vi "MWT_labview_final.vi"() -> ()   [LabVIEW 2019]
uses:
  <vilib>/BLE/type_def/connection_status_bundle.ctl
  <vilib>/BLE/type_def/address_type.ctl
  <vilib>/BLE/ble_functions/ble_write_by_service_characteristic_uint8array.vi
panel:
  out "characteristic value":u8[](array[numeric])
  in  "transmission inteveral (Seconds)":u8[](array[numeric]) format="%02x"
  out "Gradient graph":dbl(graph)
  out "Gradient":dbl
  out "VDD":dbl
  out "Temperature graph":dbl(graph)
  out "Temperature":dbl
  out "Rotation graph":dbl(graph)
  out "Rotation Speed":dbl
  in  "stop":bool
  out "Reading data":bool
  out "Connected":bool
  out "Device Name":string
  out "Handle table":string[][](array[string])
  out "Connection Status":T1={"MAC Address"="", "cnx handle"=0, "cnx flags"=0, "Address Type"=125, "Connection Interval (ms)"=125, "Timeout(ms)"=125, "Latency"=0, "bonding handle"=0} {"Address Type" items=["Public", "Random"]}
  out "Scanning":bool
  in  "COM Bluegiga in":refnum<visa-resource-name>="COM13"
  out "Devices":string[][](array[string])
  out "BLED112 Dongle Info":string
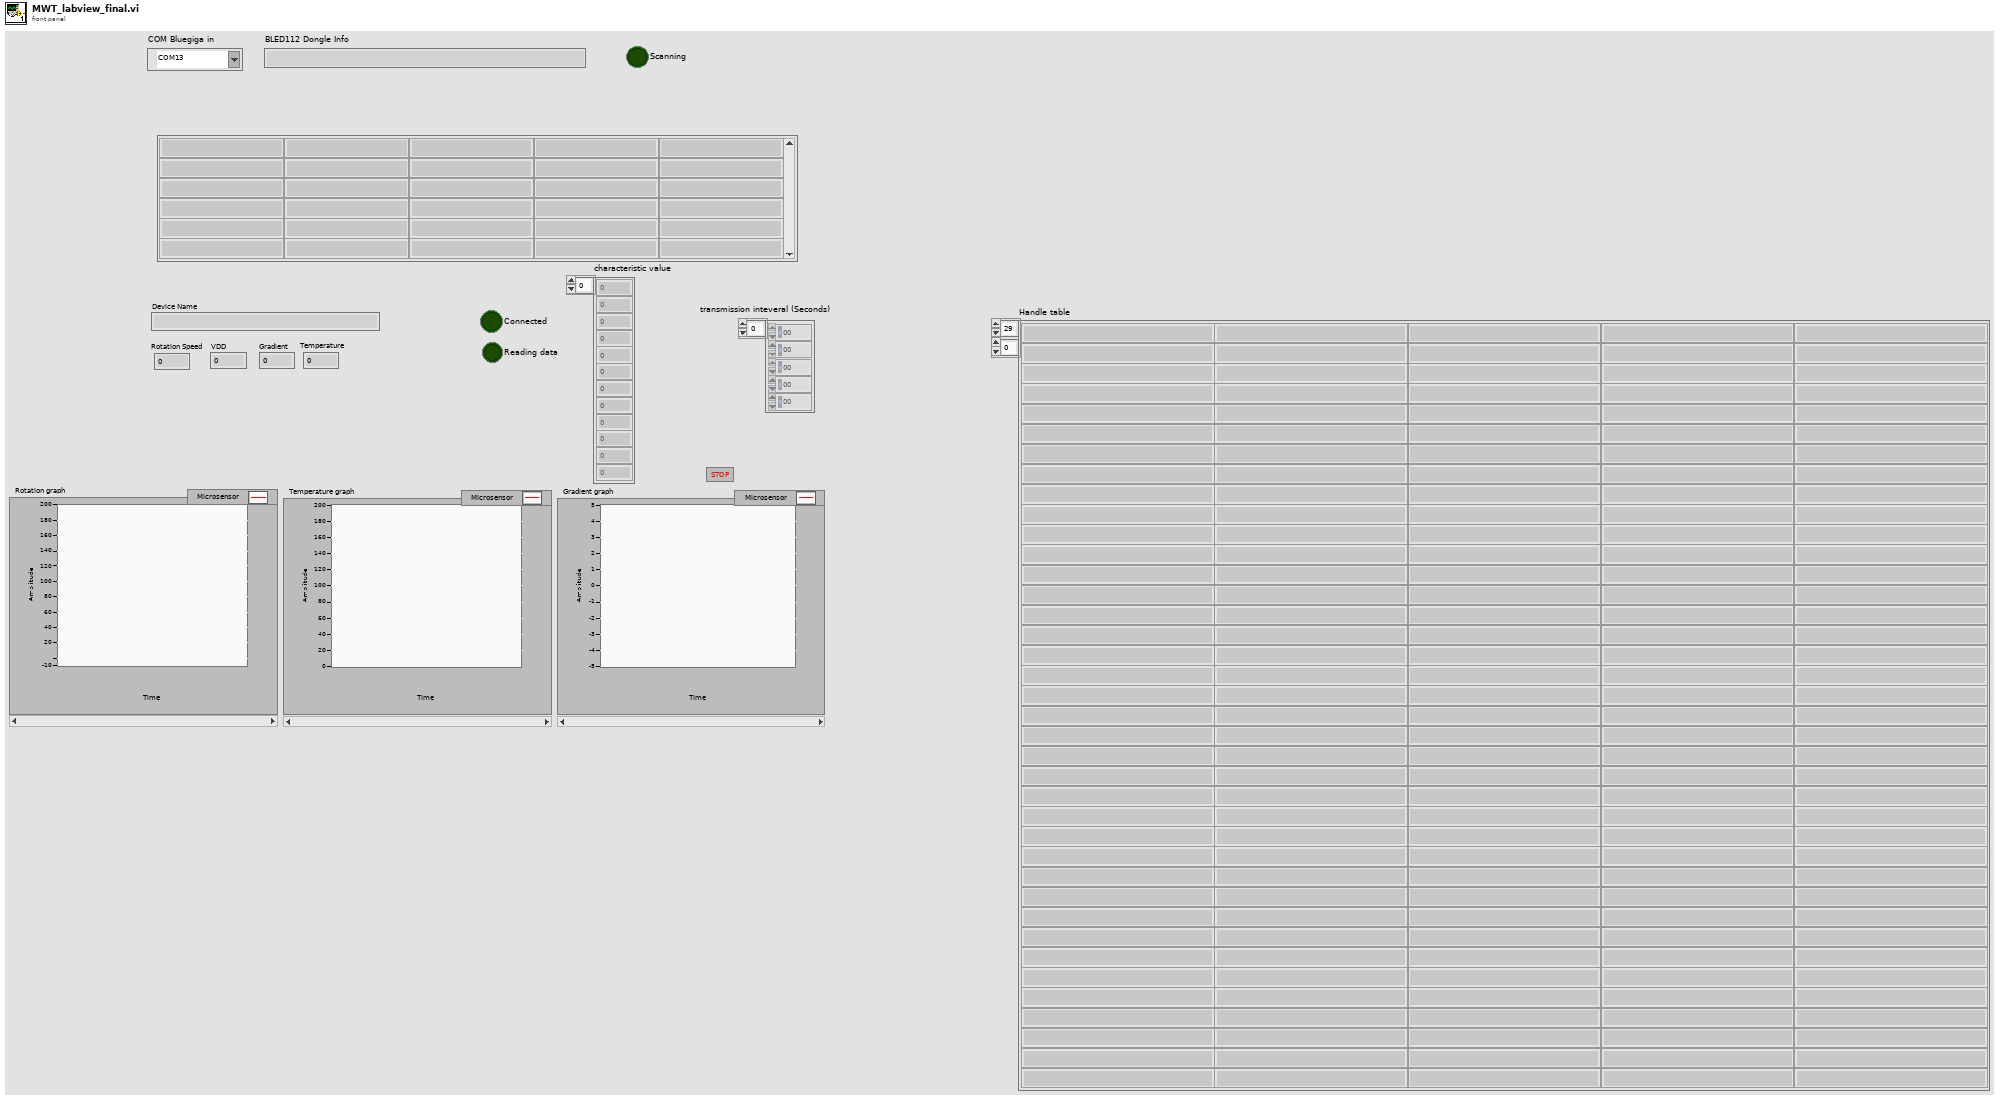
[diagram p1: front panel]
types:
  T1 = typedef "connection_status_bundle.ctl" = cluster{"MAC Address":string, "cnx handle":u8, "cnx flags":u8, "Address Type":T2, "Connection Interval (ms)":u16, "Timeout(ms)":u16, "Latency":u16, "bonding handle":u8}
  T2 = typedef "address_type.ctl" = u8
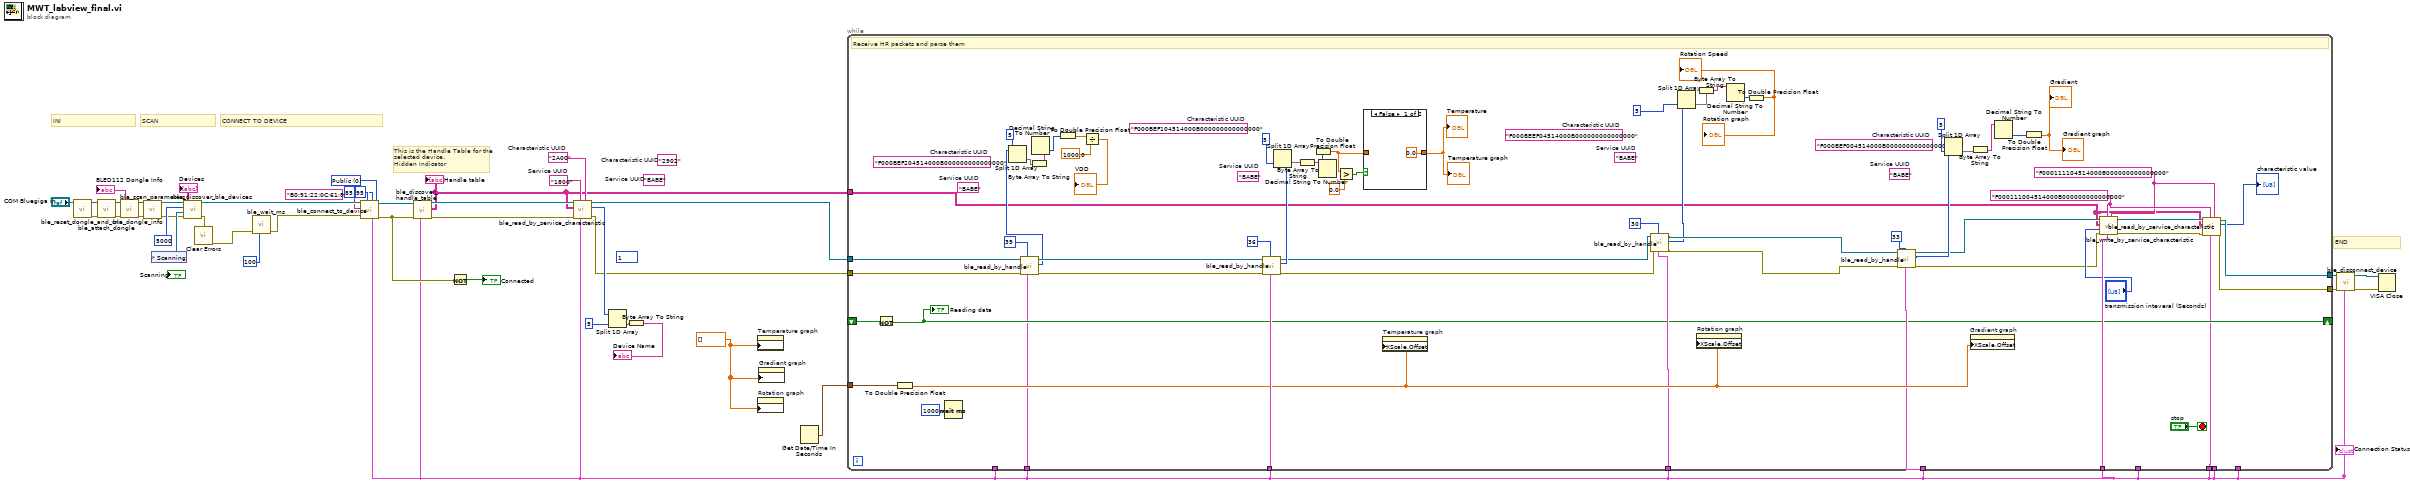
[diagram p0: block diagram]
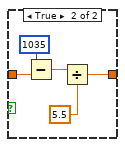
[diagram p2: hidden frame]
diagram:
  w14 = T2 0 items=["Public", "Random"] ("Address Type")
  w12 = dbl[] [] ("History Data")
  (unwired) "2902"  # Characteristic UUID
  (unwired) "BABE"  # Service UUID
  (unwired) u16 1 ("Value(16bit)")
  w21 = "2A00"  # Characteristic UUID
  w22 = "1800"  # Service UUID
  # "END"
  # "This is the Handle Table for the\nselected device. \nHidden Indicator"
  # "CONNECT TO DEVICE"
  # "SCAN"
  # "INI"
  n1 = call <vilib>:"ble_reset_dongle_and_cnx.vi"("COM Bluegiga in"="COM Bluegiga in") -> ("error out"=w33:errorcluster, "COM Bluegiga out"=w31:refnum<visa-resource-name>)  [unwired: 9 in]
  n2 = call <vilib>:"ble_attach_dongle.vi"("error in (no error)"=w33, "COM Bluegiga in"=w31) -> ("error out"=w35:errorcluster, "COM Bluegiga out"=w34:refnum<visa-resource-name>)  [unwired: 8 in]
  n3 = call <vilib>:"ble_dongle_info.vi"("error in (no error)"=w35, "COM Bluegiga in"=w34) -> ("error out"=w38:errorcluster, "info"=→"BLED112 Dongle Info":string, "COM Bluegiga out"=w39:refnum<visa-resource-name>)  [unwired: 7 in]
  n4 = call <vilib>:"ble_scan_parameters.vi"("error in (no error)"=w38, "COM Bluegiga in"=w39) -> ("error out"=w36:errorcluster, "COM Bluegiga out"=w37:refnum<visa-resource-name>)  [unwired: 7 in, 1 out]
  n5 = control-ref of="Scanning"() -> (w40:refnum<vi>)
  n6 = call <vilib>:"ble_discover_ble_devices.vi"("error in (no error)"=w36, "LED ref"=w40, "Scan Duration (10000ms)"=u32 5000, "COM Bluegiga in"=w37) -> ("error out"=w29:errorcluster, "Devices"=→"Devices":string[][], "COM Bluegiga out"=w15:refnum<visa-resource-name>)  [unwired: 5 in]
  n7 = call <vilib>:"Clear Errors.vi"("error in (no error)"=w29) -> ("error out"=w18:errorcluster)  [unwired: 5 in, 1 out]
  n8 = call <vilib>:"ble_wait_ms.vi"("milliseconds to wait (100)"=u32 100, "error in (no error)"=w18) -> ("error out"=w17:errorcluster)  [unwired: 9 in]
  n9 = call <vilib>:"ble_connect_to_device.vi"("Address Type"=w14, "Connection Interval Max (95ms)"=u16 95, "Connection Interval Min (75ms)"=u16 85, "error in (no error)"=w17, "MAC Address"="B0:91:22:0C:61:84", "COM Bluegiga in"=w15) -> ("error out"=w23:errorcluster, "COM Bluegiga out"=w30:refnum<visa-resource-name>, "Connection Status"=w2:T1)  [unwired: 3 in]
  "Connection Status" <- w2
  n10 = call <vilib>:"ble_discover_handle_table.vi"("Connection Status"=w2, "error in (no error)"=w23, "COM Bluegiga in"=w30) -> ("error out"=w28:errorcluster, "Handle table"=w1:string[][], "COM Bluegiga out"=w27:refnum<visa-resource-name>)  [unwired: 6 in]
  "Handle table" <- w1
  n11 = Not(x=w23) -> (.not. x?=→"Connected":bool)
  n12 = call <vilib>:"ble_read_by_service_characteristic.vi"("Characteristic UUID"=w21, "Connection Status"=w2, "Service UUID"=w22, "error in (no error)"=w28, "Handle table"=w1, "COM Bluegiga in"=w27) -> ("error out"=w5:errorcluster, "characteristic value"=w20:u8[], "COM Bluegiga out"=w6:refnum<visa-resource-name>)  [unwired: 3 in]
  n13 = Split 1D Array(array=w20, index=5) -> (second subarray=w19:u8[])  [unwired: 1 out]
  n14 = Byte Array To String(unsigned byte array=w19) -> (string=→"Device Name":string)
  n15 = property on="Temperature graph" class="WFChart (strict)"("History Data"=w12) -> ()  [unwired: 2 in, 2 out]
  n16 = property on="Rotation graph" class="WFChart (strict)"("History Data"=w12) -> ()  [unwired: 2 in, 2 out]
  n17 = property on="Gradient graph" class="WFChart (strict)"("History Data"=w12) -> ()  [unwired: 2 in, 2 out]
  n18 = Get Date/Time In Seconds() -> (seconds since 1Jan1904=w9:timestamp)
  n19 = while {
    shift-right: [w68] -> _
    shift-left: _ -> [w106]
    tunnel: w2 -> [w72]
    tunnel: w2 -> [w95]
    tunnel: w2 -> [_]
    tunnel: w2 -> [w70]
    tunnel: w9 -> [w78]
    tunnel: w2 -> [_]
    tunnel: w2 -> [w76]
    tunnel: w6 -> [w64]
    tunnel: w5 -> [w63]
    tunnel: w2 -> [w62]
    tunnel: w2 -> [_]
    tunnel: w2 -> [_]
    tunnel: [w50] -> w4
    tunnel: [w49] -> w3
    tunnel: w2 -> [w45]
    tunnel: w1 -> [w44]
    stop <- "stop" stop-if-true
    w47 = "F000111004514000B000000000000000" ("Service UUID")
    w46 = "F000111104514000B000000000000000" ("Characteristic UUID")
    (unwired) "F000BEF004514000B000000000000000"  # Characteristic UUID
    (unwired) "BABE"  # Service UUID
    (unwired) "F000BEF204514000B000000000000000"  # Characteristic UUID
    (unwired) "BABE"  # Service UUID
    (unwired) "F000BEF104514000B000000000000000"  # Characteristic UUID
    (unwired) "BABE"  # Service UUID
    (unwired) "F000BEEF04514000B000000000000000"  # Characteristic UUID
    (unwired) "BABE"  # Service UUID
    # "Receive HR packets and parse them"
    n20 = Not(x=w106) -> (.not. x?=w68:bool)
    "Reading data" <- w68
    n21 = To Double Precision Float(number=w78) -> (double precision float=w79:dbl)
    n22 = Wait (ms)(milliseconds to wait=u32 1000) -> ()  [unwired: 1 out]
    n23 = call <vilib>:"ble_read_by_handle.vi"("Connection Status"=w62, "Handle"=u16 39, "error in (no error)"=w63, "COM Bluegiga in"=w64) -> ("error out"=w66:errorcluster, "characteristic value"=w61:u8[], "COM Bluegiga out"=w67:refnum<visa-resource-name>)  [unwired: 5 in]
    n24 = Split 1D Array(array=w61, index=5) -> (second subarray=w53:u8[])  [unwired: 1 out]
    n25 = Byte Array To String(unsigned byte array=w53) -> (string=w93:string)
    n26 = Decimal String To Number(string=w93) -> (number=w92:i32)  [unwired: 2 in, 1 out]
    n27 = To Double Precision Float(number=w92) -> (double precision float=w91:dbl)
    n28 = Divide(x=w91, y=1000.0) -> (x/y=→"VDD":dbl)
    n29 = call <vilib>:"ble_read_by_handle.vi"("Connection Status"=w95, "Handle"=u16 36, "error in (no error)"=w66, "COM Bluegiga in"=w67) -> ("error out"=w73:errorcluster, "characteristic value"=w96:u8[], "COM Bluegiga out"=w74:refnum<visa-resource-name>)  [unwired: 5 in]
    n30 = Split 1D Array(array=w96, index=5) -> (second subarray=w97:u8[])  [unwired: 1 out]
    n31 = Byte Array To String(unsigned byte array=w97) -> (string=w100:string)
    n32 = Decimal String To Number(string=w100) -> (number=w98:i32)  [unwired: 2 in, 1 out]
    n33 = To Double Precision Float(number=w98) -> (double precision float=w88:dbl)
    n34 = Greater?(x=w88, y=0.0) -> (0:w86:bool)
    n35 = case shown="False" w86 {
      tunnel: w88 -> [_ w113]
      tunnel: [0.0 w109] -> w85
      frame False {
      }
      frame True {
        n36 = Subtract(x=1035, y=w113) -> (x-y=w110:dbl)
        n37 = Divide(x=w110, y=5.5) -> (x/y=w109:dbl)
      }
    }
    "Temperature" <- w85
    "Temperature graph" <- w85
    n38 = property on="Temperature graph" class="WFChart (strict)"("XScale.Offset"=w79) -> ()  [unwired: 2 in, 2 out]
    n39 = call <vilib>:"ble_read_by_handle.vi"("Connection Status"=w72, "Handle"=u16 30, "error in (no error)"=w73, "COM Bluegiga in"=w74) -> ("error out"=w59:errorcluster, "characteristic value"=w58:u8[], "COM Bluegiga out"=w60:refnum<visa-resource-name>)  [unwired: 5 in]
    n40 = Split 1D Array(array=w58, index=5) -> (second subarray=w104:u8[])  [unwired: 1 out]
    n41 = property on="Rotation graph" class="WFChart (strict)"("XScale.Offset"=w79) -> ()  [unwired: 2 in, 2 out]
    n42 = Byte Array To String(unsigned byte array=w104) -> (string=w103:string)
    n43 = Decimal String To Number(string=w103) -> (number=w102:i32)  [unwired: 2 in, 1 out]
    n44 = To Double Precision Float(number=w102) -> (double precision float=→"Rotation Speed" →"Rotation graph":dbl)
    n45 = call <vilib>:"ble_read_by_handle.vi"("Connection Status"=w70, "Handle"=u16 33, "error in (no error)"=w59, "COM Bluegiga in"=w60) -> ("error out"=w54:errorcluster, "characteristic value"=w56:u8[], "COM Bluegiga out"=w55:refnum<visa-resource-name>)  [unwired: 5 in]
    n46 = Split 1D Array(array=w56, index=5) -> (second subarray=w83:u8[])  [unwired: 1 out]
    n47 = property on="Gradient graph" class="WFChart (strict)"("XScale.Offset"=w79) -> ()  [unwired: 2 in, 2 out]
    n48 = Byte Array To String(unsigned byte array=w83) -> (string=w82:string)
    n49 = Decimal String To Number(string=w82) -> (number=w81:i32)  [unwired: 2 in, 1 out]
    n50 = To Double Precision Float(number=w81) -> (double precision float=→"Gradient" →"Gradient graph":dbl)
    n51 = call-poly <vilib>:"ble_write_by_service_characteristic.vi"("Characteristic UUID"=w46, "Connection Status"=w76, "Service UUID"=w47, "error in (no error)"=w54, "data"="transmission inteveral (Seconds)", "Handle table"=w44, "COM Bluegiga in"=w55) -> ("error out"=w51:errorcluster, "COM Bluegiga out"=w52:refnum<visa-resource-name>)  [unwired: 3 in]
    n52 = call <vilib>:"ble_read_by_service_characteristic.vi"("Characteristic UUID"=w46, "Connection Status"=w45, "Service UUID"=w47, "error in (no error)"=w51, "Handle table"=w44, "COM Bluegiga in"=w52) -> ("error out"=w49:errorcluster, "characteristic value"=→"characteristic value":u8[], "COM Bluegiga out"=w50:refnum<visa-resource-name>)  [unwired: 3 in]
  }
  n53 = call <vilib>:"ble_disconnect_device.vi"("Connection Status"=w2, "error in (no error)"=w3, "COM Bluegiga in"=w4) -> ("error out"=w10:errorcluster, "COM Bluegiga out"=w11:refnum<visa-resource-name>)  [unwired: 7 in]
  n54 = VISA Close(VISA resource name=w11, error in (no error)=w10) -> ()  [unwired: 1 out]
